vi "FTW-Request-Receive.vi"(5 "MessagePipe":refnum<queue>, 11 "error in":errorcluster) -> (4 "Request":refnum<data-value>, 6 "Request Header":string, 15 "error out":errorcluster)   [LabVIEW 2015]
uses:
  json/core/FTW-JSON-Core-Structure.ctl
  error/FTW-ERR-ThrowError.vi
  error/FTW-ERR-CallChain.vi
  error/FTW-ERR-NoErrorConstant.vi
  string/FTW-STR-ReplaceWhitespace.vi
  string/FTW-STR-Array-Delimit.vi
  error/FTW-ERR-Clear.vi
  regex/FTW-Regex-ReplaceAll.vi
panel:
  # "Inputs"
  # "Outputs"
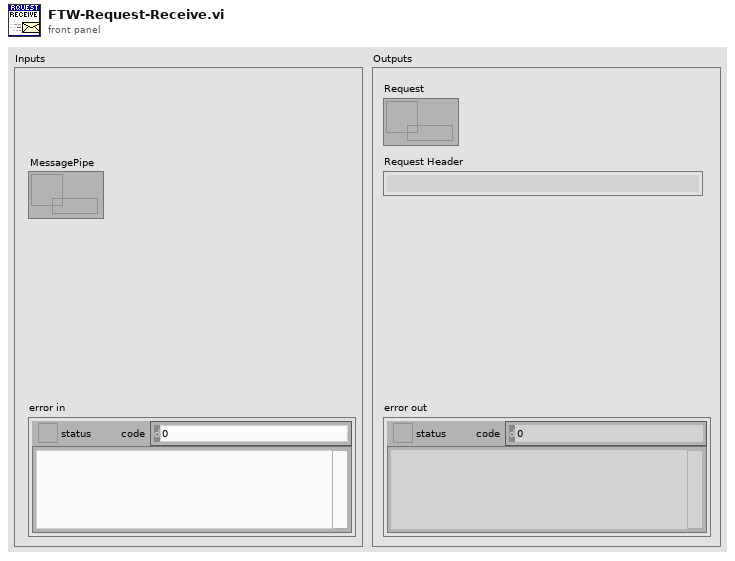
[diagram p1: front panel]
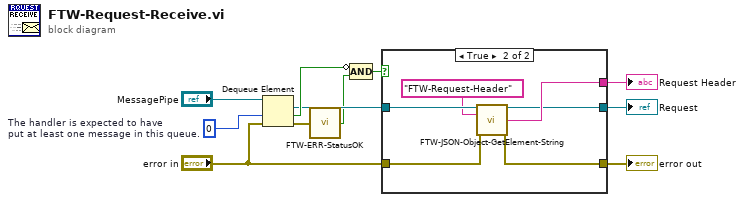
[diagram p0: block diagram]
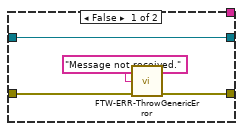
[diagram p2: hidden frame]
diagram:
  w8 = 0  # The handler is expected to have put at least one message in this queue.
  n1 = Dequeue Element(queue="MessagePipe", timeout in ms (-1)=w8, error in (no error)="error in") -> (element=w5:refnum<data-value>, timed out?=w6:bool, error out=w4:errorcluster)  [unwired: 1 out]
  n2 = call "FTW-ERR-StatusOK.vi"("error to check"=w4) -> ("Status OK?"=w3:bool)
  n3 = Compound Arithmetic op=AND(invert w6, w3) -> (w2:bool)
  n4 = case shown="True" w2 {
    tunnel: [w14 w16] -> w9
    tunnel: [_ w21] -> w11
    tunnel: [w12 w18] -> w10
    tunnel: w5 -> [w12 w20]
    tunnel: "error in" -> [w13 w17]
    frame False {
      n5 = call "FTW-ERR-ThrowGenericError.vi"("Error Message"="Message not received.", "error in"=w13) -> ("error out"=w14:errorcluster)  [unwired: 13 in]
    }
    frame True {
      n6 = call "FTW-JSON-Object-GetElement-String.vi"("JSON Object"=w20, "Key"="FTW-Request-Header", "error in"=w17) -> ("JSON Object out"=w18:refnum<data-value>, "Value"=w21:string, "error out"=w16:errorcluster)  [unwired: 9 in, 1 out]
    }
  }
  "error out" <- w9
  "Request Header" <- w11
  "Request" <- w10
